vi "Load_from_Project.vi"(8 "error in (no error)":errorcluster, 9 "index":i32, 10 "buildObject":T3, 11 "AB_Source_RESTfulVI in":refnum<class "AB_Source_RESTfulVI.lvclass">) -> (0 "error out":errorcluster, 2 "linker info":T2, 3 "AB_Source_RESTfulVI out":refnum<class "AB_Source_RESTfulVI.lvclass">)   [LabVIEW 2020, in "AB_Source_RESTfulVI.lvclass"]
uses:
  <vilib>/AppBuilder/AB_Classes/Source/RESTfulVI/AB_Source_RESTfulVI.lvclass
  <resource>/Framework/Providers/API/ItemRef.ctl
  <vilib>/Utility/lvfile.llb/LVFileType.ctl
  <vilib>/AppBuilder/RW_Project/AB_RW_Project_PropBag_Action.ctl
  <vilib>/AppBuilder/AB_Classes/Source/RESTfulVI/AB_Source_RESTfulVI.lvclass/AB_Source_RESTfulVI.ctl
  <vilib>/AppBuilder/AB_Classes/Source/VI/AB_Source_VI.lvclass
  <vilib>/Utility/lvfile.llb/NI_FileType.lvlib
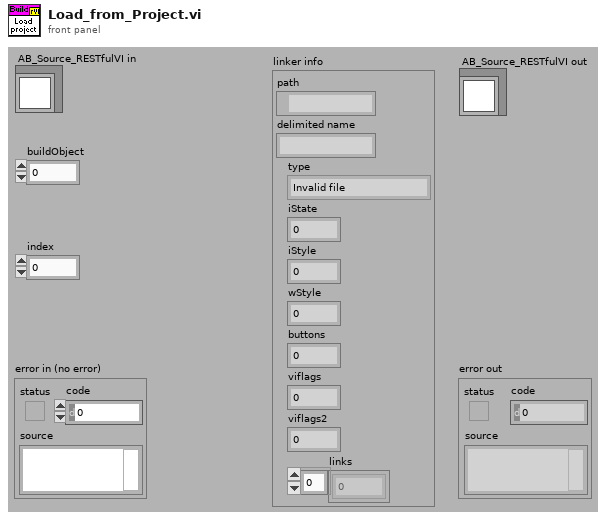
[diagram p1: front panel]
types:
  T1 = typedef "NI_FileType.lvlib/LVFileType.ctl" = enum32{"Invalid file", "Unknown type", "Instrument", "Control", "Polymorphic VI", "Project", "Library", "LVClass", "XControl", "XNode", "Shared library", ".NET assembly", "ActiveX interface", "CIN", "Run-time menu", "Palette menu", "Help file", "LLB", "XNode Edit Dependency", "Class Private Data Control", "Statechart", "MathScript .m file", "Ladder Diagram", "LVLibp", "XNode Build Dependency"}
  T2 = cluster{"path":path, "delimited name":string, "type":T1, "iState":u32, "iStyle":u16, "wStyle":u16, "buttons":u16, "viflags":u32, "viflags2":u32, "links":u32[]}
  T3 = typedef "ItemRef.ctl" = u64
  T4 = typedef "AB_RW_Project_PropBag_Action.ctl" = enum16{"read", "write", "clear", "readPrevious", "writePrevious", "clearPrevious"}
  T5 = typedef "AB_RW_Project_Source_RESTfulVI_Data.ctl" = cluster{"RESTful VI configuration":T6}
  T6 = typedef "AB_RESTful_Configuration.ctl" = cluster{"Service VI Type":T7, "Load VI at statup":bool, "Keep VI in memory":bool, "Output type":T8, "Output format":T9, "Use headers":bool, "Buffered":bool, "eng_Load VI by name":bool}
  T7 = typedef "AB_RESTful_VIType.ctl" = enum32{"Web Method", "Auxiliary", "eng_Internal", "eng_Content"}
  T8 = typedef "AB_RESTful_OutputType.ctl" = enum32{"Terminal", "Stream"}
  T9 = typedef "AB_RESTful_OutputFormat.ctl" = enum32{"XML", "Text", "HTML", "JSON"}
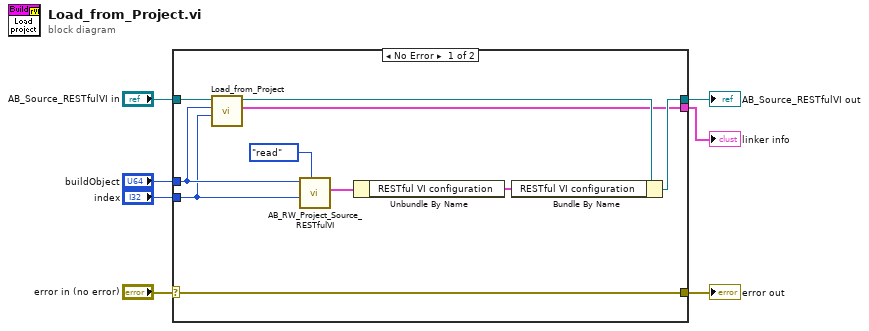
[diagram p0: block diagram]
diagram:
  n1 = case shown="No Error" "error in (no error)" {
    selector: "error in (no error)" -> [w16 w18]
    tunnel: "AB_Source_RESTfulVI in" -> [w17 w19]
    tunnel: [w11 w19] -> w5
    tunnel: [w16 w18] -> w4
    tunnel: "buildObject" -> [w15 _]
    tunnel: "index" -> [w14 _]
    tunnel: [w8 _] -> w1
    frame No Error {
      n2 = call-parent "Load_from_Project.vi"("index"=w14, "buildObject"=w15, "AB_Source_VI in"=w17) -> ("linker info"=w8:T2, "AB_Source_VI out"=w12:refnum<class "AB_Source_RESTfulVI.lvclass">)  [unwired: 6 in, 1 out]
      n3 = call <vilib>:"AB_RW_Project_Source_RESTfulVI.vi"("action"=AB_RW_Project_PropBag_Action."read", "index in"=w14, "buildObject"=w15) -> ("dataSource out"=w10:T5)  [unwired: 5 in, 3 out]
      n4 = Unbundle By Name(w10) -> ("RESTful VI configuration"=w9:T6)
      n5 = Bundle By Name(cluster=w12, "RESTful VI configuration"=w9) -> (w11:refnum<class "AB_Source_RESTfulVI.lvclass">)
    }
    frame Error {
    }
  }
  "error out" <- w4
  "AB_Source_RESTfulVI out" <- w5
  "linker info" <- w1
